vi "Update Data.vi"(8 "error in (no error)":errorcluster, 10 "Debug Data":refnum<class "Debug Data.lvclass">[](array[class]), 11 "List Seen Processes View Model In":refnum<class "List Processes View Model.lvclass">) -> (0 "error out":errorcluster, 3 "List Seen Processes View Model Out":refnum<class "List Processes View Model.lvclass">)   [LabVIEW 2020, in "List Processes View Model.lvclass"]
uses:
  List Processes View Model.lvclass
  C:/Git/astemes-triarc-debugger/source/List Box View Model_/List Box View Model.lvclass
  Debug Data/Debug Data.lvclass
  Debug Data/Debug Data.lvclass/Debug Data.ctl
  List Box View Model_/List Box View Model.lvclass/List Box View Model.ctl
  List Processes View Model.lvclass/List Processes View Model.ctl
  List Box View Model_/List Box View Model.lvclass
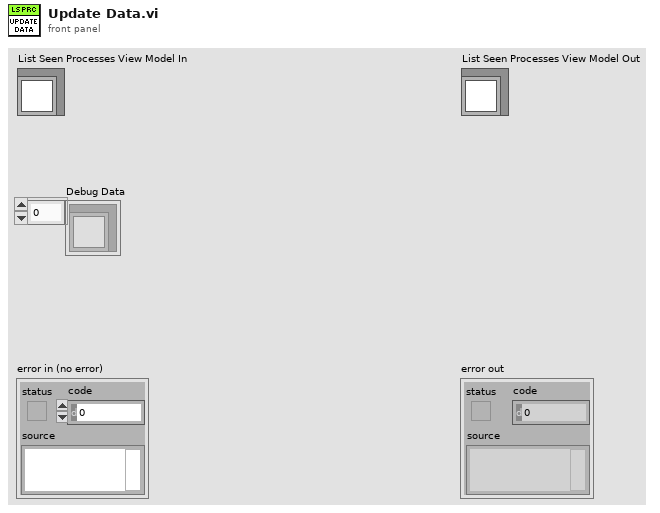
[diagram p1: front panel]
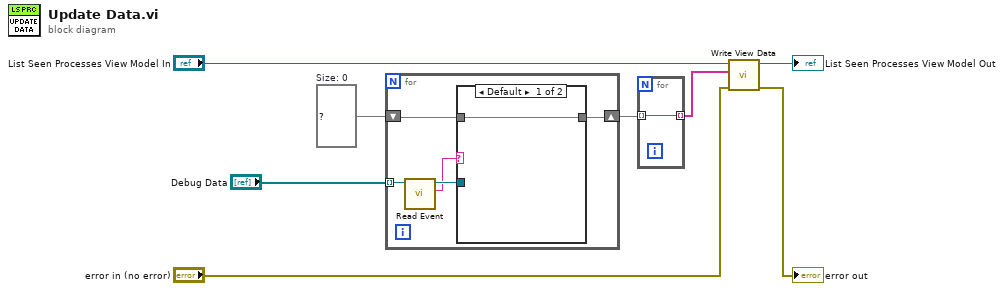
[diagram p0: block diagram]
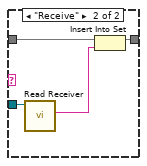
[diagram p2: hidden frame]
diagram:
  w6 = set{string} {}  # Size: 0
  n1 = for {
    tunnel: "Debug Data" -> [w13] mode=indexing
    shift-right: [w11] -> w2
    shift-left: w6 -> [w12]
    n2 = call "Read Event.vi"("Debug Data in"=w13) -> ("Event"=w9:string, "Debug Data out"=w10:refnum<class "Debug Data.lvclass">)  [unwired: 9 in]
    n3 = case shown="Default" w9 {
      tunnel: w12 -> [w14 w18]
      tunnel: [w14 w16] -> w11
      tunnel: w10 -> [_ w15]
      frame Default {
      }
      frame "Receive" {
        n4 = call "Read Receiver.vi"("Debug Data In"=w15) -> ("Receiver"=w17:string)  [unwired: 9 in, 1 out]
        n5 = Insert Into Set(10:w17, 11:w18) -> (3:w16:set{string})  [unwired: 1 out]
      }
    }
  }
  n6 = for {
    tunnel: [w19] -> w1 mode=indexing
    tunnel: w2 -> [w19] mode=indexing
  }
  n7 = call "Write View Data.vi"("error in (no error)"="error in (no error)", "View Data"=w1, "List Box View Model In"="List Seen Processes View Model In") -> ("error out"=→"error out":errorcluster, "List Box View Model Out"=→"List Seen Processes View Model Out":refnum<class "List Processes View Model.lvclass">)  [unwired: 7 in]
